vi "Flow Ranges.vi"() -> (0 "Flow Ranges":dbl[unit][](array[numeric])=[2.221666666666667e-06, 2.2216666666666667e-05, 0.00022216666666666668, 0.002221666666666667, 0.002221666666666667, 0.02221666666666667, 0.22216666666666668, 2.2216666666666667, 2.2216666666666667, 22.21666666666667, 222.16666666666669, 1.6666666666666669e-06, 1.6666666666666667e-05, 0.0001666666666666667, 0.0016666666666666668, 0.0016666666666666668, 0.016666666666666666, 0.16666666666666669, 1.6666666666666667, 1.6666666666666667, 16.666666666666668, 166.66666666666669, 1.6666666666666667e-05, 0.0001666666666666667, 0.0016666666666666668, 0.016666666666666666, 0.16666666666666669, 1.6666666666666667, 16.666666666666668])   [LabVIEW 2016, in "MGC647C.lvlib"]
doc: "This VI provides full scale flow ranges supported by the instrument."
uses:
  MGC647C.lvlib
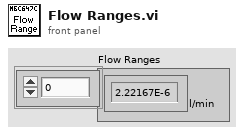
[diagram p1: front panel]
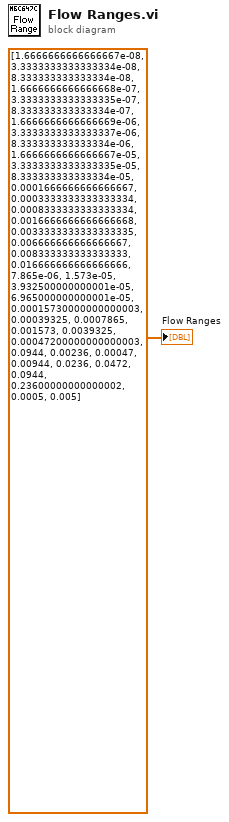
[diagram p0: block diagram]
diagram:
  "Flow Ranges" <- dbl[unit][] [1.6666666666666667e-08, 3.3333333333333334e-08, 8.333333333333334e-08, 1.6666666666666668e-07, 3.3333333333333335e-07, 8.333333333333334e-07, 1.6666666666666669e-06, 3.3333333333333337e-06, 8.333333333333334e-06, 1.6666666666666667e-05, 3.3333333333333335e-05, 8.333333333333334e-05, 0.0001666666666666667, 0.0003333333333333334, 0.0008333333333333334, 0.0016666666666666668, 0.0033333333333333335, 0.006666666666666667, 0.008333333333333333, 0.016666666666666666, 7.865e-06, 1.573e-05, 3.932500000000001e-05, 6.965000000000001e-05, 0.00015730000000000003, 0.00039325, 0.0007865, 0.001573, 0.0039325, 0.00047200000000000003, 0.0944, 0.00236, 0.00047, 0.00944, 0.0236, 0.0472, 0.0944, 0.23600000000000002, 0.0005, 0.005] ("array")
